vi "SubROIDesp.vi"(11 "Array":i16[](array[numeric])) -> (3 "output cluster":T1)   [LabVIEW 2015]
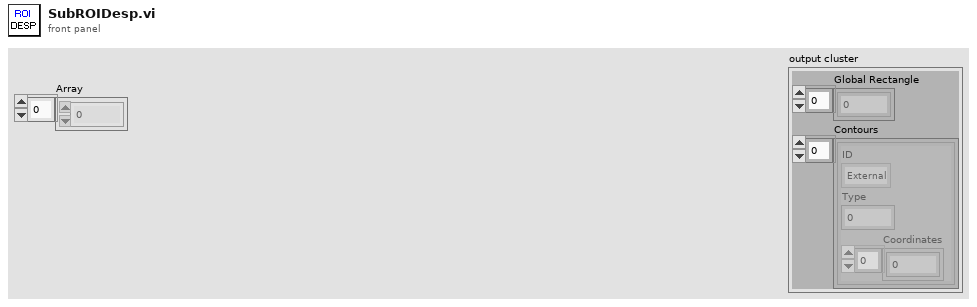
[diagram p1: front panel]
types:
  T1 = cluster{"Global Rectangle":i32[], "Contours":cluster{"ID":enum32{"External", "Internal"}, "Type":u32, "Coordinates":i32[]}[]}
  T2 = cluster{"ID":enum32{"External", "Internal"}, "Type":u32, "Coordinates":i32[]}[]
  T3 = cluster{"ID":enum32{"External", "Internal"}, "Type":u32, "Coordinates":i32[]}
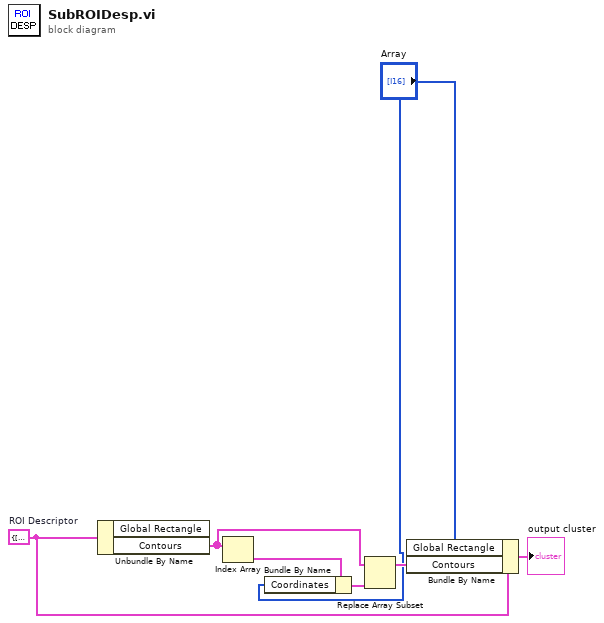
[diagram p0: block diagram]
diagram:
  w2 = T1 {"Global Rectangle"=[20, 20, 1909, 1070], "Contours"=[{"ID"=enum."External", "Type"=3, "Coordinates"=[20, 20, 1909, 1070]}]}  # ROI Descriptor
  n1 = Unbundle By Name(w2) -> ("Contours"=w4:T2)  [unwired: 1 out]
  n2 = Index Array(array=w4) -> (element=w3:T3)  [unwired: 1 in]
  n3 = Bundle By Name(cluster=w3, "Coordinates"="Array") -> (w6:T3)
  n4 = Replace Array Subset(array=w4, new element=w6) -> (w7:T2)  [unwired: 1 in]
  n5 = Bundle By Name(cluster=w2, "Global Rectangle"="Array", "Contours"=w7) -> (→"output cluster":T1)
